vi "Load Config.vi"(8 "error in (no error)":errorcluster, 11 "BridgeChannel in":refnum<class "BridgeChannel.lvclass">) -> (0 "error out":errorcluster, 3 "BridgeChannel out":refnum<class "BridgeChannel.lvclass">)   [LabVIEW 2023, in "VolatusDAQConfig.lvlib" / "BridgeChannel.lvclass"]
uses:
  BridgeChannel.lvclass
  VolatusConfig/VolatusConfigElement/VolatusConfigElement.lvclass/VolatusConfigElement.ctl
  BridgeChannel.lvclass/BridgeChannel.ctl
  VolatusConfig/VolatusConfigElement/Element.vi
  VolatusConfig/VolatusConfigElement/VolatusConfigElement.lvclass
  lv-cdm/CDM-Config/Config Element/Config Element.lvclass
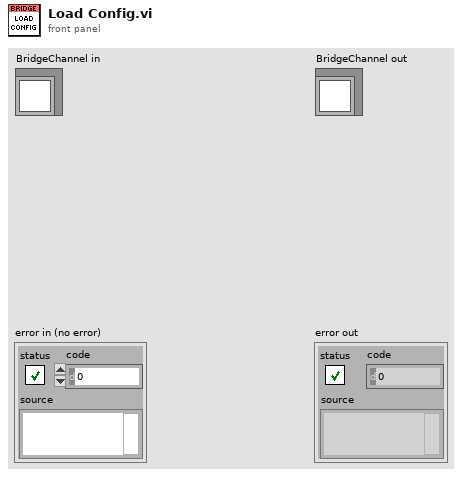
[diagram p1: front panel]
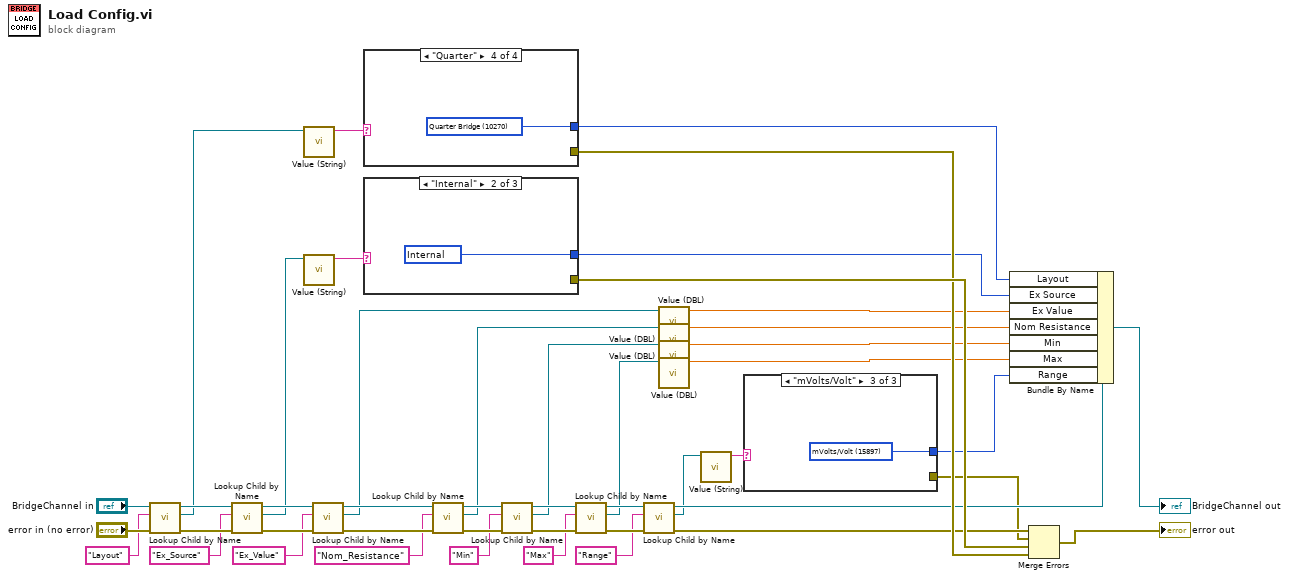
[diagram p0: block diagram]
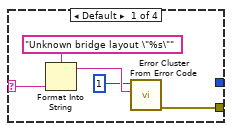
[diagram p2: hidden frame]
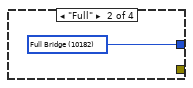
[diagram p3: hidden frame]
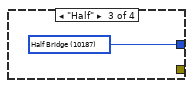
[diagram p4: hidden frame]
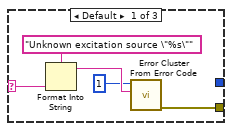
[diagram p5: hidden frame]
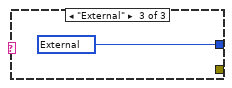
[diagram p6: hidden frame]
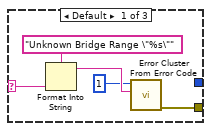
[diagram p7: hidden frame]
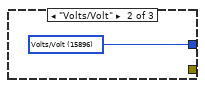
[diagram p8: hidden frame]
diagram:
  n1 = call "Lookup Child by Name.vi"("error in (no error)"="error in (no error)", "Child Name"="Layout", "VolatusConfigElement in"="BridgeChannel in") -> ("error out"=w41:errorcluster, "Child"=w1:refnum<class "Config Element.lvclass">, "VolatusConfigElement out"=w37:refnum<class "BridgeChannel.lvclass">)  [unwired: 5 in, 1 out]
  n2 = call "Lookup Child by Name.vi"("error in (no error)"=w41, "Child Name"="Ex_Source", "VolatusConfigElement in"=w37) -> ("error out"=w38:errorcluster, "Child"=w6:refnum<class "Config Element.lvclass">, "VolatusConfigElement out"=w34:refnum<class "BridgeChannel.lvclass">)  [unwired: 5 in, 1 out]
  n3 = call "Value (String).vi"("Config Element in"=w1) -> ("String Value"=w3:string)  [unwired: 9 in, 1 out]
  n4 = call "Value (String).vi"("Config Element in"=w6) -> ("String Value"=w5:string)  [unwired: 9 in, 1 out]
  n5 = call "Lookup Child by Name.vi"("error in (no error)"=w38, "Child Name"="Ex_Value", "VolatusConfigElement in"=w34) -> ("error out"=w35:errorcluster, "Child"=w7:refnum<class "Config Element.lvclass">, "VolatusConfigElement out"=w31:refnum<class "BridgeChannel.lvclass">)  [unwired: 5 in, 1 out]
  n6 = case shown="\"Quarter\"" w3 {
    selector: w3 -> [w50 _ _ _]
    tunnel: [_ w51 w52 w53] -> w2
    tunnel: [w46 _ _ _] -> w44
    frame Default {
      n7 = Format Into String(format string="Unknown bridge layout \"%s\"", w50) -> (resulting string=w48:string)  [unwired: 2 in, 1 out]
      n8 = call <vilib>:"Error Cluster From Error Code.vi"("error message (\"\")"=w48, "error code (0)"=1) -> ("error out"=w46:errorcluster)  [unwired: 7 in]
    }
    frame "Full" {
      w51 = 10182 items=["Full Bridge"=10182, "Half Bridge"=10187, "Quarter Bridge"=10270] ("Layout")
    }
    frame "Half" {
      w52 = 10187 items=["Full Bridge"=10182, "Half Bridge"=10187, "Quarter Bridge"=10270] ("Layout")
    }
    frame "Quarter" {
      w53 = 10270 items=["Full Bridge"=10182, "Half Bridge"=10187, "Quarter Bridge"=10270] ("Layout")
    }
  }
  n9 = case shown="\"Internal\"" w5 {
    selector: w5 -> [w58 _ _]
    tunnel: [_ w59 w60] -> w4
    tunnel: [w54 _ _] -> w45
    frame Default {
      n10 = Format Into String(format string="Unknown excitation source \"%s\"", w58) -> (resulting string=w56:string)  [unwired: 2 in, 1 out]
      n11 = call <vilib>:"Error Cluster From Error Code.vi"("error message (\"\")"=w56, "error code (0)"=1) -> ("error out"=w54:errorcluster)  [unwired: 7 in]
    }
    frame "Internal" {
      w59 = 10200 items=["Internal"=10200, "External"=10167] ("Ex Source")
    }
    frame "External" {
      w60 = 10167 items=["Internal"=10200, "External"=10167] ("Ex Source")
    }
  }
  n12 = call "Lookup Child by Name.vi"("error in (no error)"=w35, "Child Name"="Nom_Resistance", "VolatusConfigElement in"=w31) -> ("error out"=w32:errorcluster, "Child"=w8:refnum<class "Config Element.lvclass">, "VolatusConfigElement out"=w28:refnum<class "BridgeChannel.lvclass">)  [unwired: 5 in, 1 out]
  n13 = call "Lookup Child by Name.vi"("error in (no error)"=w32, "Child Name"="Min", "VolatusConfigElement in"=w28) -> ("error out"=w29:errorcluster, "Child"=w9:refnum<class "Config Element.lvclass">, "VolatusConfigElement out"=w25:refnum<class "BridgeChannel.lvclass">)  [unwired: 5 in, 1 out]
  n14 = call "Lookup Child by Name.vi"("error in (no error)"=w29, "Child Name"="Max", "VolatusConfigElement in"=w25) -> ("error out"=w26:errorcluster, "Child"=w10:refnum<class "Config Element.lvclass">, "VolatusConfigElement out"=w23:refnum<class "BridgeChannel.lvclass">)  [unwired: 5 in, 1 out]
  n15 = call "Lookup Child by Name.vi"("error in (no error)"=w26, "Child Name"="Range", "VolatusConfigElement in"=w23) -> ("error out"=w17:errorcluster, "Child"=w20:refnum<class "Config Element.lvclass">, "VolatusConfigElement out"=w22:refnum<class "BridgeChannel.lvclass">)  [unwired: 5 in, 1 out]
  n16 = call "Value (DBL).vi"("Config Element in"=w7) -> ("DBL Value"=w11:dbl)  [unwired: 9 in, 1 out]
  n17 = call "Value (DBL).vi"("Config Element in"=w8) -> ("DBL Value"=w12:dbl)  [unwired: 9 in, 1 out]
  n18 = call "Value (DBL).vi"("Config Element in"=w9) -> ("DBL Value"=w13:dbl)  [unwired: 9 in, 1 out]
  n19 = call "Value (DBL).vi"("Config Element in"=w10) -> ("DBL Value"=w14:dbl)  [unwired: 9 in, 1 out]
  n20 = call "Value (String).vi"("Config Element in"=w20) -> ("String Value"=w19:string)  [unwired: 9 in, 1 out]
  n21 = case shown="\"mVolts/Volt\"" w19 {
    selector: w19 -> [w65 _ _]
    tunnel: [_ w66 w67] -> w18
    tunnel: [w61 _ _] -> w16
    frame Default {
      n22 = Format Into String(format string="Unknown Bridge Range \"%s\"", w65) -> (resulting string=w63:string)  [unwired: 2 in, 1 out]
      n23 = call <vilib>:"Error Cluster From Error Code.vi"("error message (\"\")"=w63, "error code (0)"=1) -> ("error out"=w61:errorcluster)  [unwired: 7 in]
    }
    frame "Volts/Volt" {
      w66 = 15896 items=["Volts/Volt"=15896, "mVolts/Volt"=15897, "From Custom Scale"=10065] ("units")
    }
    frame "mVolts/Volt" {
      w67 = 15897 items=["Volts/Volt"=15896, "mVolts/Volt"=15897, "From Custom Scale"=10065] ("units")
    }
  }
  n24 = Bundle By Name(cluster=w22, "Layout"=w2, "Ex Source"=w4, "Ex Value"=w11, "Nom Resistance"=w12, "Min"=w13, "Max"=w14, "Range"=w18) -> (→"BridgeChannel out":refnum<class "BridgeChannel.lvclass">)
  n25 = Merge Errors(w17, w16, w45, w44) -> (→"error out":errorcluster)
